vi "Axsun Queue Manager.vi"(5 "queue name":enum16{"Axsun processor", "Axsun GUI"}(ring)=enum."Axsun GUI", 6 "timeout in ms (-1)":i32=-1, 7 "Action":T1=enum."Enqueue", 8 "Error In":errorcluster, 11 "Message Packet Array":T2[](array[typedef])) -> (0 "Error Out":errorcluster, 1 "Empty?":bool, 2 "# elements in queue":i32, 3 "Message Packet [Out]":T2)   [LabVIEW 2018]
uses:
  Controls/MessagePacket.ctl
  Controls/Queue Manager Actions.ctl
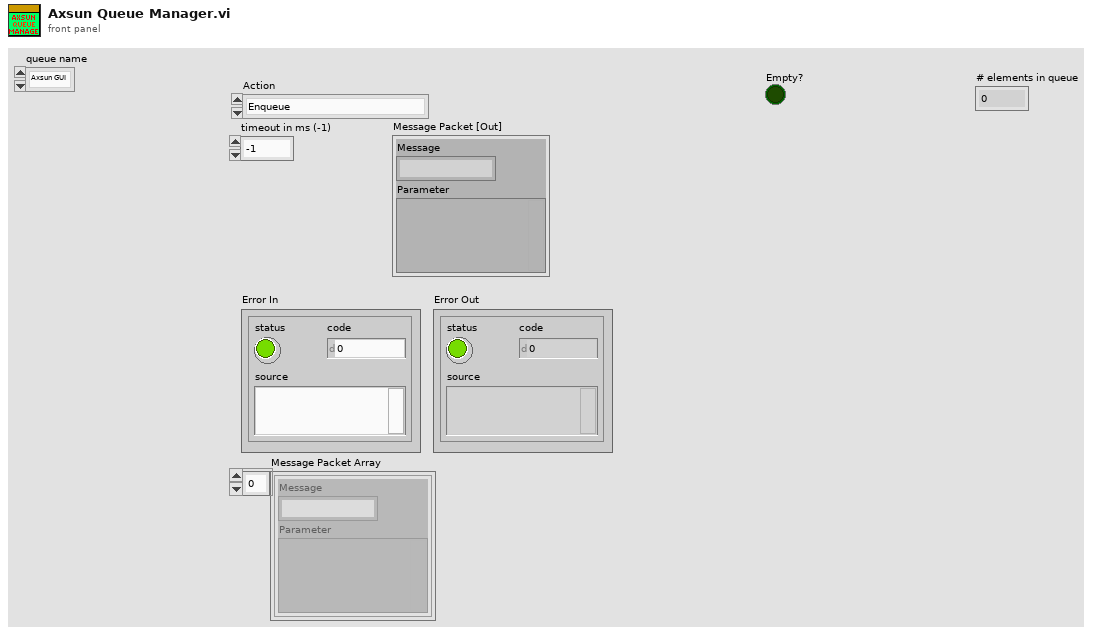
[diagram p1: front panel]
types:
  T1 = typedef "Queue Manager Actions.ctl" = enum16{"Init", "Enqueue", "Enqueue All", "Preview Queue", "Dequeue", "Get Status", "Flush Queue", "Flush All Queues", "Release All Queues", "Release Queue", "Enqueue at Opposite End"}
  T2 = typedef "MessagePacket.ctl" = cluster{"Message":string, "Parameter":variant}
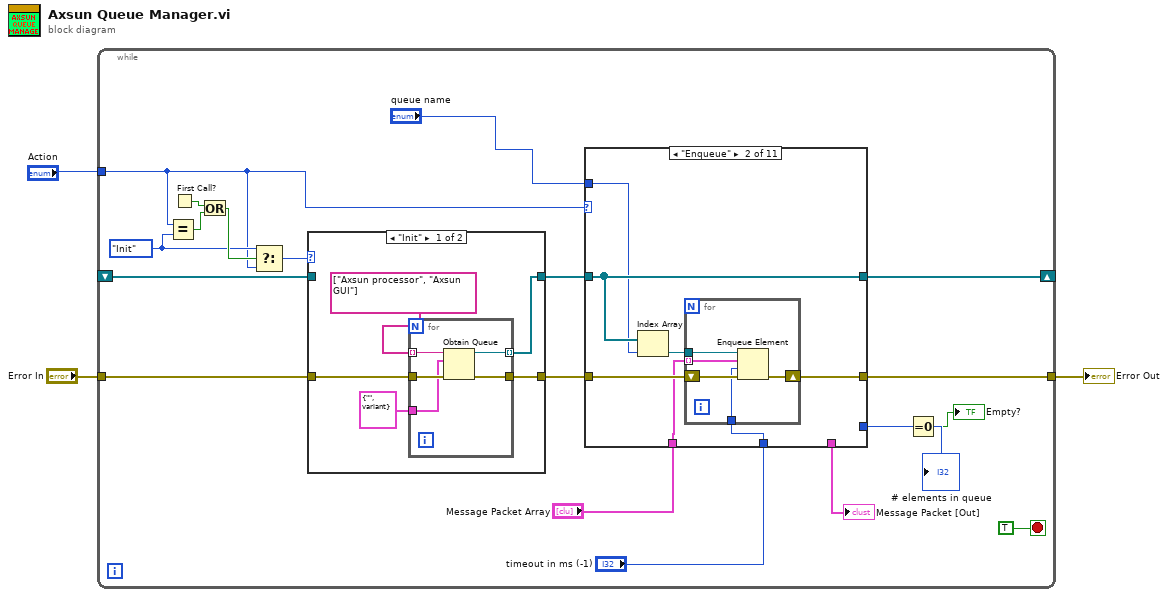
[diagram p0: block diagram]
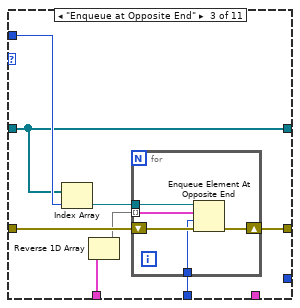
[diagram p3: hidden frame]
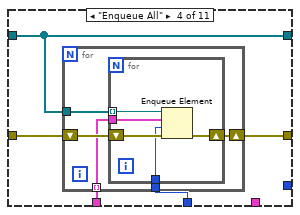
[diagram p4: hidden frame]
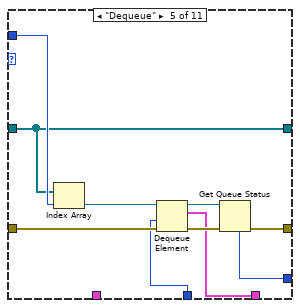
[diagram p5: hidden frame]
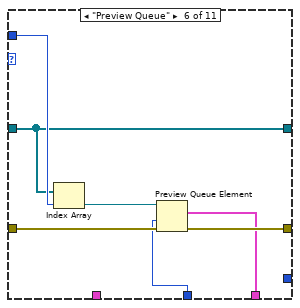
[diagram p6: hidden frame]
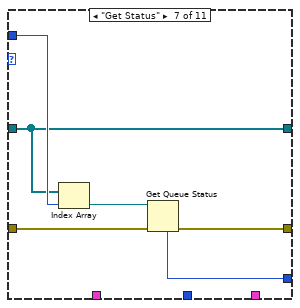
[diagram p7: hidden frame]
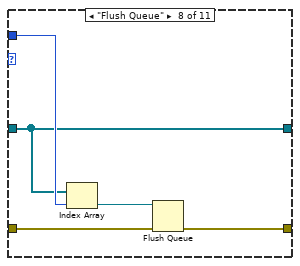
[diagram p8: hidden frame]
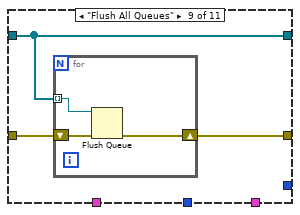
[diagram p9: hidden frame]
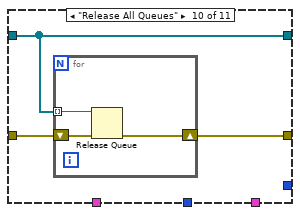
[diagram p10: hidden frame]
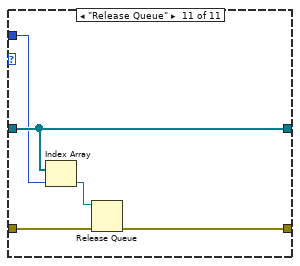
[diagram p11: hidden frame]
diagram:
  n1 = while {
    tunnel: "Action" -> [w8]
    tunnel: "Error In" -> [w17]
    tunnel: [w16] -> w1
    shift-right: [w10] -> _
    shift-left: _ -> [w9]
    stop <- TRUE stop-if-true
    w19 = Queue_Manager_Actions."Init"
    n2 = Equal?(x=w8, y=w19) -> (x = y?=w21:bool)
    n3 = First Call?() -> (First Call?: T/F=w22:bool)
    n4 = Or(x=w22, y=w21) -> (x .or. y?=w20:bool)
    n5 = Select(t=w19, s=w20, f=w8) -> (s? t:f=w18:T1)
    n6 = case shown="\"Init\"" w18 {
      tunnel: [w114 w120] -> w14
      tunnel: w17 -> [w113 w121]
      tunnel: [w112 w121] -> w15
      tunnel: w9 -> [_ w120]
      frame "Init" {
        n7 = for {
          tunnel: string[] ["Axsun processor", "Axsun GUI"] -> [w115] mode=indexing
          tunnel: [w119] -> w114 mode=indexing
          tunnel: w113 -> [w118]
          tunnel: [w117] -> w112
          tunnel: T2 {"Message"="", "Parameter"=variant} ("Message Packet") -> [w116]
          n8 = Obtain Queue(name (unnamed)=w115, element data type=w116, error in (no error)=w118) -> (queue out=w119:refnum<queue>, error out=w117:errorcluster)  [unwired: 2 in, 1 out]
        }
      }
      frame "Enqueue", Default {
      }
    }
    n9 = case shown="\"Enqueue\"" w8 {
      tunnel: w14 -> [w23 w27 w39 w51 w65 w76 w83 w88 w93 w99 w107]
      tunnel: [w24 w30 w43 w53 w68 w80 w86 w89 w94 w100 w108] -> w16
      tunnel: w15 -> [w24 w31 w44 w54 w74 w81 w87 w92 w95 w101 w109]
      tunnel: "queue name" -> [_ w25 w42 _ w72 w79 w85 w91 _ _ w106]
      tunnel: "Message Packet Array" -> [_ w28 w40 w52 _ _ _ _ _ _ _]
      tunnel: [_ _ _ _ w70 w77 _ _ _ _ _] -> w13
      tunnel: [w23 w27 w39 w51 w65 w76 w83 w88 w93 w99 w107] -> w10
      tunnel: "timeout in ms (-1)" -> [_ w26 w37 w50 w69 w75 _ _ _ _ _]
      tunnel: [_ _ _ _ w66 _ w82 _ _ _ _] -> w6
      frame "Init", Default {
      }
      frame "Enqueue" {
        n10 = Index Array(array=w27, index=w25) -> (element=w29:refnum<queue>)
        n11 = for {
          tunnel: w29 -> [w34]
          tunnel: w28 -> [w33] mode=indexing
          shift-right: [w35] -> w30
          shift-left: w31 -> [w36]
          tunnel: w26 -> [w32]
          n12 = Enqueue Element(queue=w34, element=w33, timeout in ms (-1)=w32, error in (no error)=w36) -> (error out=w35:errorcluster)  [unwired: 2 out]
        }
      }
      frame "Enqueue at Opposite End" {
        n13 = Index Array(array=w39, index=w42) -> (element=w41:refnum<queue>)
        n14 = Reverse 1D Array(array=w40) -> (reversed array=w38:T2[])
        n15 = for {
          tunnel: w41 -> [w47]
          tunnel: w38 -> [w46] mode=indexing
          shift-right: [w48] -> w43
          shift-left: w44 -> [w49]
          tunnel: w37 -> [w45]
          n16 = Enqueue Element At Opposite End(queue=w47, element=w46, timeout in ms (-1)=w45, error in (no error)=w49) -> (error out=w48:errorcluster)  [unwired: 2 out]
        }
      }
      frame "Enqueue All" {
        n17 = for {
          tunnel: w52 -> [w57] mode=indexing
          shift-right: [w58] -> w53
          shift-left: w54 -> [w59]
          tunnel: w51 -> [w56]
          tunnel: w50 -> [w55]
          n18 = for {
            tunnel: w56 -> [w62] mode=indexing
            tunnel: w57 -> [w61]
            shift-right: [w63] -> w58
            shift-left: w59 -> [w64]
            tunnel: w55 -> [w60]
            n19 = Enqueue Element(queue=w62, element=w61, timeout in ms (-1)=w60, error in (no error)=w64) -> (error out=w63:errorcluster)  [unwired: 2 out]
          }
        }
      }
      frame "Dequeue" {
        n20 = Index Array(array=w65, index=w72) -> (element=w71:refnum<queue>)
        n21 = Dequeue Element(queue=w71, timeout in ms (-1)=w69, error in (no error)=w74) -> (queue out=w67:refnum<queue>, element=w70:T2, error out=w73:errorcluster)  [unwired: 1 out]
        n22 = Get Queue Status(queue=w67, error in (no error)=w73) -> (error out=w68:errorcluster, # elements in queue=w66:i32)  [unwired: 1 in, 6 out]
      }
      frame "Preview Queue" {
        n23 = Index Array(array=w76, index=w79) -> (element=w78:refnum<queue>)
        n24 = Preview Queue Element(queue=w78, timeout in ms (-1)=w75, error in (no error)=w81) -> (element=w77:T2, error out=w80:errorcluster)  [unwired: 2 out]
      }
      frame "Get Status" {
        n25 = Index Array(array=w83, index=w85) -> (element=w84:refnum<queue>)
        n26 = Get Queue Status(queue=w84, error in (no error)=w87) -> (error out=w86:errorcluster, # elements in queue=w82:i32)  [unwired: 1 in, 6 out]
      }
      frame "Flush Queue" {
        n27 = Index Array(array=w88, index=w91) -> (element=w90:refnum<queue>)
        n28 = Flush Queue(queue=w90, error in (no error)=w92) -> (error out=w89:errorcluster)  [unwired: 2 out]
      }
      frame "Flush All Queues" {
        n29 = for {
          shift-right: [w97] -> w94
          shift-left: w95 -> [w98]
          tunnel: w93 -> [w96] mode=indexing
          n30 = Flush Queue(queue=w96, error in (no error)=w98) -> (error out=w97:errorcluster)  [unwired: 2 out]
        }
      }
      frame "Release All Queues" {
        n31 = for {
          shift-right: [w103] -> w100
          shift-left: w101 -> [w104]
          tunnel: w99 -> [w102] mode=indexing
          n32 = Release Queue(queue=w102, error in (no error)=w104) -> (error out=w103:errorcluster)  [unwired: 1 in, 2 out]
        }
      }
      frame "Release Queue" {
        n33 = Index Array(array=w107, index=w106) -> (element=w105:refnum<queue>)
        n34 = Release Queue(queue=w105, error in (no error)=w109) -> (error out=w108:errorcluster)  [unwired: 1 in, 2 out]
      }
    }
    "Message Packet [Out]" <- w13
    "# elements in queue" <- w6
    n35 = Equal To 0?(x=w6) -> (x = 0?=→"Empty?":bool)
  }
  "Error Out" <- w1
